vi "CPA.vi"(0 "System no.":i32=1 min=1 max=4 step=1, 2 "Source":T1, 3 "Destination":T1=enum."FLASH", 5 "error in":errorcluster, 6 "Container Unit":string, 7 "Parameter ID":string, 8 "Function Unit":string) -> (19 "error out":errorcluster)   [LabVIEW 2020]
doc: "CPA (Copy Value Between Memories)\n\nDescription \nCopies values of Configuration parameters between the different memories of the \ncontroller.\n\nFormat\nCPA <SourceMemoryType> <DestinationMemoryType>[ <Container Unit>[ <Function Unit>[ \n<ParameterID>]]]\n\nArguments\n<SourceMemoryType>\nType of memory from which the values are to be copied; the \"source\"\nPossible values: RAM, TMP, FLASH\n<DestinationMemoryType>\nType of memory to which the values are to be copied; the \"destination\"\nPossible values: RAM, TMP, FLASH\n<Container Unit>\nContainer unit, whose parameter/s is/are to be copied\nThe existing container units can be queried with USG? SYS.\nPossible values: Alias of the container unit\n<Function Unit>\nFunction unit, whose parameter/s is/are to be copied\nThe existing function units can be queried with USG? SYS.\nIf a single parameter belonging to a container unit is to be copied, \"-\" must be entered for \n<Function Unit>.\nPossible values:\nAlias of the function unit\n\"-\" \n<ParameterID>\nThe value of the parameter addressed by <Container Unit>, <Function Unit> and <ParameterID> \nwill be copied to the specified memory.\n<ParameterID> always contains a parameter identifier in hexadecimal format. For 0-\ndimensional parameters, <ParameterID> is fully specified by the parameter identifier.\nFor one-dimensional and multi-dimensional parameters, an element address is also required \ntogether with the parameter identifier. Depending on the dimension of the parameter, the \nelement address consists of one or more parts that are separated from the parameter identifier \nand each other by a comma.\n- One-dimensional parameter (vector) -> the element address is ,number\n- Two-dimensional parameter (two-dimensional matrix) -> the element address is \n,number,number\n- Three-dimensional parameter (three-dimensional matrix) -> the element address \nis ,number,number,number\nThe address data for the parameters can be queried with USG? PAM. \nPossible values:\n0x0000 to 0xFFFF\nFor one-dimensional and multi-dimensional parameters, an additional integer >= 1 for each \ndimension\n\nResponse\nnone\n\nExample\nThe parameter 0x110 of SYS_1 TRSF_1 in the following examples forms a two-dimensional \nmatrix in the format 4x2.\n>> CPA TMP RAM\n>> CPA TMP RAM SYS_1\n>> CPA TMP RAM SYS_1 TRSF_1\n>> CPA TMP RAM SYS_1 TRSF_1 0x110\n>> CPA TMP RAM SYS_1 TRSF_1 0x110,4,2\n\nNotes\nUsing the USG? PAM command, the available parameters and their properties can be queried. \nThe response includes amongst other things the user command level for the write access \n(<WRITE-UCL> column) to the parameter value. The UCL? command (p. 71) queries the active \nuser command level. Use the UCL command (p. 69) to change to the appropriate user command \nlevel.\nThe value of a parameter can be read from the different memories of the controller using the \nSPV? command. \nThe SPV command can be used to set the values of Configuration parameters in the \ndifferent memories of the controller.\nFor further details, see \"Parameter Handling - GCS 3.0\". \n\nUser command level\nUSR"
uses:
  ConfigurationMemoryType.ctl
panel:
  # "CPA (Copy Value Between Memories)\n\nCopies values of Configuration parameters between the different memories of the controller."
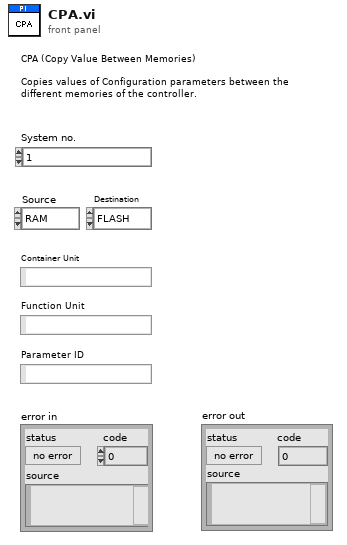
[diagram p1: front panel]
types:
  T1 = typedef "ConfigurationMemoryType.ctl" = enum16{"RAM", "TMP", "FLASH"}
  T2 = typedef "Syntax.ctl" = enum16{"GCS 1.0", "GCS 2.0", "GCS 3.0"}
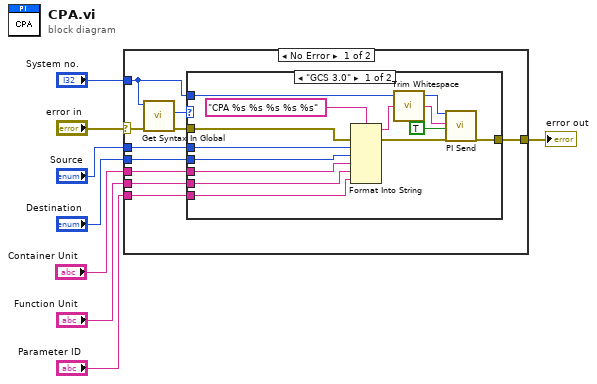
[diagram p0: block diagram]
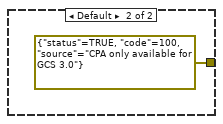
[diagram p2: hidden frame]
diagram:
  n1 = case shown="No Error" "error in" {
    selector: "error in" -> [w17 w33]
    tunnel: [w16 w33] -> w7
    tunnel: "Function Unit" -> [w12 _]
    tunnel: "Container Unit" -> [w13 _]
    tunnel: "System no." -> [w9 _]
    tunnel: "Source" -> [w15 _]
    tunnel: "Destination" -> [w14 _]
    tunnel: "Parameter ID" -> [w11 _]
    frame No Error {
      n2 = call "Get Syntax In Global.vi"("error in"=w17, "System no."=w9) -> ("error out"=w18:errorcluster, "Syntax"=w10:T2)  [unwired: 8 in]
      n3 = case shown="\"GCS 3.0\"" w10 {
        tunnel: [w20 errorcluster {"status"=TRUE, "code"=100, "source"="CPA only available for GCS 3.0"} ("error out")] -> w16
        tunnel: w18 -> [w28 _]
        tunnel: w15 -> [w31 _]
        tunnel: w14 -> [w29 _]
        tunnel: w13 -> [w27 _]
        tunnel: w12 -> [w26 _]
        tunnel: w11 -> [w25 _]
        tunnel: w9 -> [w19 _]
        frame "GCS 3.0" {
          n4 = Format Into String(format string="CPA %s %s %s %s %s", error in=w28, w31, w29, w27, w26, w25) -> (resulting string=w24:string, error out=w23:errorcluster)  [unwired: 1 in]
          n5 = call <vilib>:"Trim Whitespace.vi"("string"=w24) -> ("trimmed string"=w21:string)  [unwired: 1 in]
          n6 = call "PI Send.vi"("System no."=w19, "String to send"=w21, "Attach termination char.?"=TRUE, "error in"=w23) -> ("error out"=w20:errorcluster)  [unwired: 2 in, 13 out]
        }
        frame Default {
        }
      }
    }
    frame Error {
    }
  }
  "error out" <- w7
